vi "asdasd.vi"() -> ()   [LabVIEW 2018]
panel:
  out "decimal integer string":string
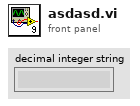
[diagram p1: front panel]
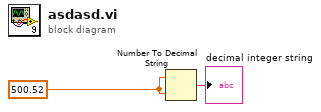
[diagram p0: block diagram]
diagram:
  w2 = 500.52
  n1 = Number To Decimal String(number=w2, width (-)=w2) -> (decimal integer string=→"decimal integer string":string)
